vi "FPGA.vi"() -> ()   [LabVIEW 2017]
uses:
  <vilib>/rvi/Emulation/niFpgaGetClockAttributes.vi
  <vilib>/rvi/Emulation/niFpgaSctlEmulationGetInTimedLoop.vi
  <vilib>/rvi/Emulation/niFpgaEmulationReportErrorSimple.vi
  <vilib>/rvi/eio/common/nirviEmuTemplateMethod_errors.vi
  <vilib>/rvi/Emulation/niFpgaCriticalErrorInLSC.vi
  <vilib>/rvi/Emulation/niFpgaProcessEmulError.vi
  <vilib>/eio/EIONode/EIONode.xnode
panel:
  out "LOW_PRESSURE":bool
  out "ACTIVE":bool
  in  "lower lim":fxp<+/-,32,10>=1.0
  in  "upper lim":fxp<+/-,32,10>=99.0
  in  "pedal sig -> eco %":fxp<+/-,38,12>=0.75
  in  "pedal offset":fxp<+/-,37,11>=-20.0
  in  "min pressure":fxp<+/-,16,5>=1.2001953125
  out "Pedal tilt %":fxp<+/-,37,11>
  out "Pressure_regulator":fxp<+/-,64,44>
  out "WSUW":bool
  out "WYSUW":bool
  in  "ECO":bool
  out "Pedal_tilt":fxp<+/-,20,5>
  out "Piston_position":fxp<+/-,20,5>
  out "Pressure":fxp<+/-,20,5>
  out "Counts":u64
  # "CONFIG"
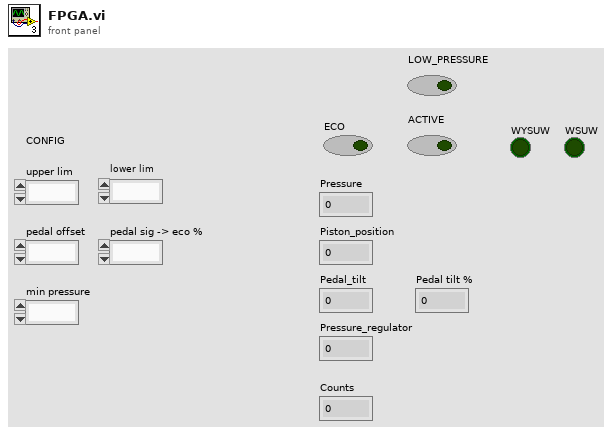
[diagram p1: front panel]
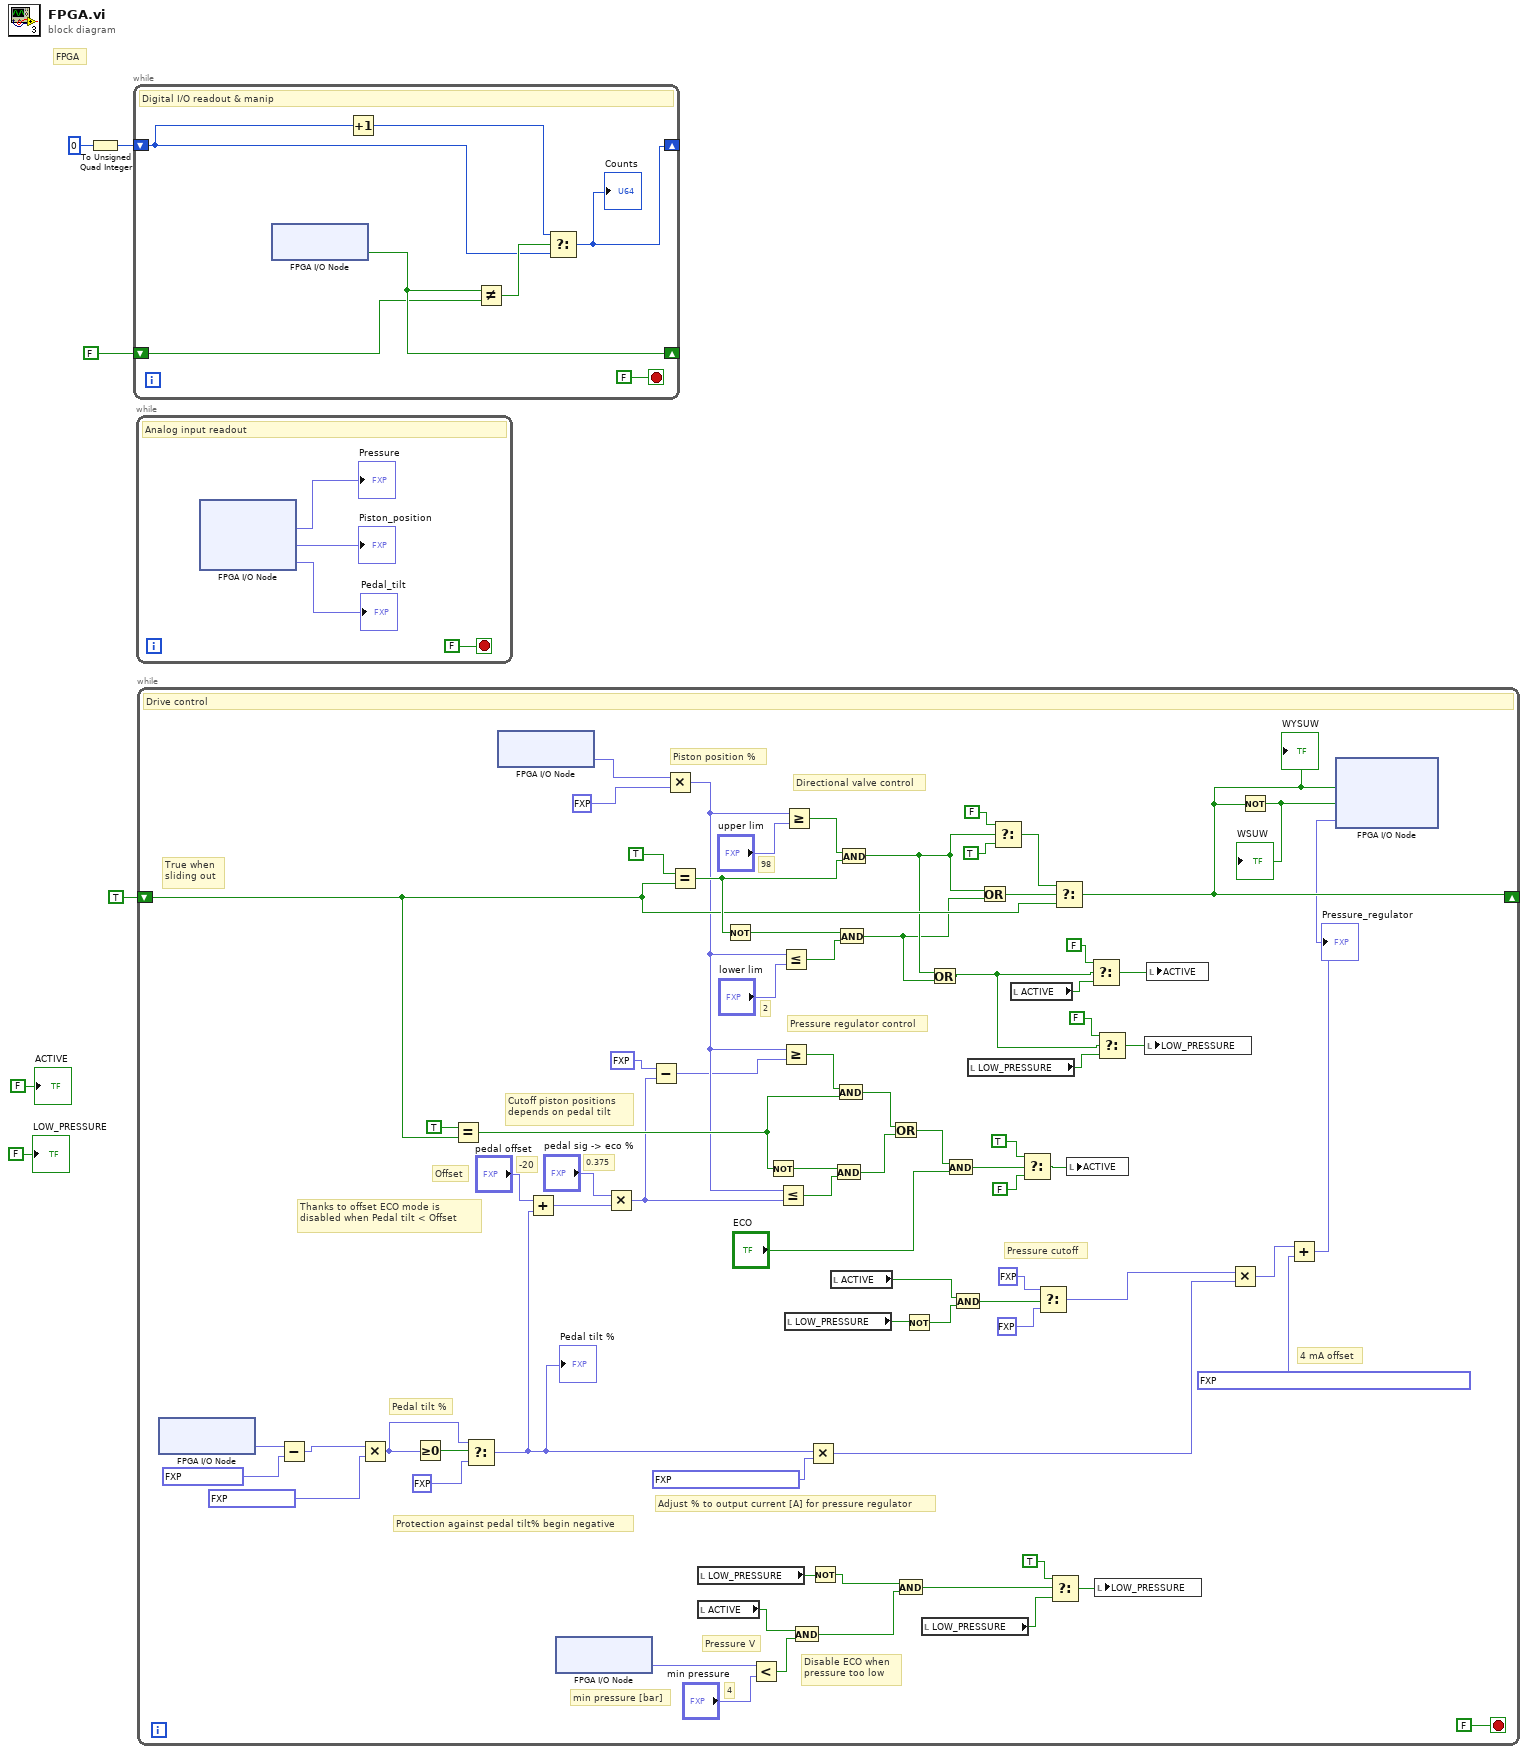
[diagram p0: block diagram]
diagram:
  # "FPGA"
  n1 = To Unsigned Quad Integer(1:i16 0) -> (0:w5:u64)
  n2 = while {
    shift-right: [w12] -> _
    shift-left: FALSE ("Mod2/DI0") -> [w11]
    shift-right: [w7] -> _
    shift-left: w5 -> [w8]
    stop <- FALSE stop-if-true
    # "Digital I/O readout & manip"
    n3 = xnode "FPGA I/O Node"() -> ("Mod2/DI0"=w12:bool)  [unwired: 1 in, 1 out]
    n4 = Increment(x=w8) -> (x+1=w9:u64)
    n5 = Not Equal?(x=w12, y=w11) -> (x != y?=w10:bool)
    n6 = Select(t=w9, s=w10, f=w8) -> (s? t:f=w7:u64)
    "Counts" <- w7
  }
  n7 = while {
    stop <- FALSE stop-if-true
    # "Analog input readout"
    n8 = xnode "FPGA I/O Node"() -> ("Mod1/AI0"=→"Pressure":fxp<+/-,16,5>, "Mod1/AI1"=→"Piston_position":fxp<+/-,16,5>, "Mod1/AI2"=→"Pedal_tilt":fxp<+/-,16,5>)  [unwired: 3 in, 3 out]
  }
  n9 = while {
    shift-right: [w78] -> _
    shift-left: TRUE -> [w79]
    stop <- FALSE stop-if-true
    # "4"
    # "2"
    # "98"
    # "0.375"
    # "-20"
    # "4 mA offset"
    # "Adjust % to output current [A] for pressure regulator"
    # "Protection against pedal tilt% begin negative"
    # "min pressure [bar]"
    # "Pressure V"
    # "Disable ECO when\npressure too low"
    # "True when sliding out"
    # "Pressure cutoff"
    # "Thanks to offset ECO mode is disabled when Pedal tilt < Offset"
    # "Offset"
    # "Cutoff piston positions\ndepends on pedal tilt"
    # "Pressure regulator control"
    # "Directional valve control"
    # "Pedal tilt %"
    # "Piston position %"
    # "Drive control"
    n10 = xnode "FPGA I/O Node"() -> ("Mod1/AI2"=w71:fxp<+/-,16,5>)  [unwired: 1 in, 1 out]
    n11 = Subtract(x=w71, y=fxp<+/-,16,5> 0.72021484375) -> (x-y=w69:fxp<+/-,17,6>)
    n12 = Multiply(x=w69, y=fxp<+/-,17,6> 25.77294921875) -> (x*y=w60:fxp<+/-,33,11>)
    n13 = Greater Or Equal To 0?(x=w60) -> (x >= 0?=w61:bool)
    n14 = Equal?(x=TRUE, y=w79) -> (x = y?=w82:bool)
    n15 = Select(t=w60, s=w61, f=fxp<+/-,37,11> 0.0) -> (s? t:f=w59:fxp<+/-,37,11>)
    "Pedal tilt %" <- w59
    n16 = xnode "FPGA I/O Node"() -> ("Mod1/AI1"=w73:fxp<+/-,16,5>)  [unwired: 1 in, 1 out]
    n17 = Add(x="pedal offset", y=w59) -> (x+y=w62:fxp<+/-,38,12>)
    n18 = xnode "FPGA I/O Node"() -> ("Mod1/AI0"=w65:fxp<+/-,16,5>)  [unwired: 1 in, 1 out]
    n19 = Multiply(x="pedal sig -> eco %", y=w62) -> (x*y=w66:fxp<+/-,64,23>)
    n20 = Subtract(x=fxp<+/-,64,23> 100.0, y=w66) -> (x-y=w75:fxp<+/-,64,24>)
    n21 = Multiply(x=w73, y=fxp<+/-,16,5> 10.0) -> (x*y=w77:fxp<+/-,32,10>)
    n22 = Equal?(x=TRUE, y=w79) -> (x = y?=w93:bool)
    n23 = local read "LOW_PRESSURE"() -> (w30:bool)
    n24 = local read "ACTIVE"() -> (w41:bool)
    n25 = Not(x=w93) -> (.not. x?=w92:bool)
    n26 = Less?(x=w65, y="min pressure") -> (x < y?=w74:bool)
    n27 = Not(x=w82) -> (.not. x?=w85:bool)
    n28 = Less Or Equal?(x=w77, y=w66) -> (x <= y?=w84:bool)
    n29 = Less Or Equal?(x=w77, y="lower lim") -> (x <= y?=w44:bool)
    n30 = Greater Or Equal?(x=w77, y=w75) -> (x >= y?=w86:bool)
    n31 = Greater Or Equal?(x=w77, y="upper lim") -> (x >= y?=w45:bool)
    n32 = local read "LOW_PRESSURE"() -> (w23:bool)
    n33 = And(x=w41, y=w74) -> (x .and. y?=w28:bool)
    n34 = Multiply(x=w59, y=fxp<+/-,33,11> 0.00015997886657714844) -> (x*y=w25:fxp<+/-,64,21>)
    n35 = Not(x=w30) -> (.not. x?=w29:bool)
    n36 = local read "ACTIVE"() -> (w24:bool)
    n37 = And(x=w85, y=w84) -> (x .and. y?=w81:bool)
    n38 = And(x=w86, y=w82) -> (x .and. y?=w36:bool)
    n39 = And(x=w92, y=w44) -> (x .and. y?=w18:bool)
    n40 = And(x=w45, y=w93) -> (x .and. y?=w19:bool)
    n41 = Or(x=w36, y=w81) -> (x .or. y?=w87:bool)
    n42 = And(x=w29, y=w28) -> (x .and. y?=w27:bool)
    n43 = Not(x=w23) -> (.not. x?=w22:bool)
    n44 = local read "LOW_PRESSURE"() -> (w26:bool)
    n45 = Or(x=w19, y=w18) -> (x .or. y?=w37:bool)
    n46 = And(x=w87, y="ECO") -> (x .and. y?=w31:bool)
    n47 = And(x=w24, y=w22) -> (x .and. y?=w21:bool)
    n48 = local read "LOW_PRESSURE"() -> (w35:bool)
    n49 = Or(x=w19, y=w18) -> (x .or. y?=w91:bool)
    n50 = Select(t=FALSE, s=w19, f=TRUE) -> (s? t:f=w88:bool)
    n51 = local read "ACTIVE"() -> (w32:bool)
    n52 = Select(t=TRUE, s=w31, f=FALSE) -> (s? t:f=w48:bool)
    n53 = Select(t=fxp<+/-,64,23> 0.0 ("x"), s=w21, f=fxp<+/-,64,23> 1.0) -> (s? t:f=w20:fxp<+/-,64,23>)
    n54 = Select(t=TRUE, s=w27, f=w26) -> (s? t:f=w39:bool)
    n55 = Select(t=w88, s=w91, f=w79) -> (s? t:f=w78:bool)
    "WYSUW" <- w78
    n56 = local write "ACTIVE"(w48) -> ()
    n57 = Select(t=FALSE, s=w37, f=w32) -> (s? t:f=w42:bool)
    n58 = local write "LOW_PRESSURE"(w39) -> ()
    n59 = Select(t=FALSE, s=w37, f=w35) -> (s? t:f=w38:bool)
    n60 = local write "LOW_PRESSURE"(w38) -> ()
    n61 = local write "ACTIVE"(w42) -> ()
    n62 = Multiply(x=w20, y=w25) -> (x*y=w34:fxp<+/-,64,44>)
    n63 = Not(x=w78) -> (.not. x?=w80:bool)
    "WSUW" <- w80
    n64 = Add(x=w34, y=fxp<+/-,64,21> 0.004000000000019099 ("x")) -> (x+y=w56:fxp<+/-,64,45>)
    "Pressure_regulator" <- w56
    n65 = xnode "FPGA I/O Node"("Mod2/DO0"=w78, "Mod2/DO1"=w80, "Mod3/AO0"=w56) -> ()  [unwired: 3 in, 3 out]
  }
  "ACTIVE" <- FALSE ("ACTIVE")
  "LOW_PRESSURE" <- FALSE ("LOW_PRESSURE")
